vi "read correction factor.vi"(8 "error in (no error)":errorcluster, 11 "Path":path=path "C:/labview project/PSA SubVIs/temp file/trace.csv") -> (0 "error out":errorcluster, 1 "Output Array":dbl[][](array[numeric]), 2 "Number of Columns":i32, 3 "Number of Rows":i32)   [LabVIEW 2016]
doc: "Transfer N*2 (transducer factor) or N*3(limit line file) CSV file to 2D Array, output number of rows and columns as well, so in next module these information can be fomat into strings of SCPI commnad which will be written into PSA through for loop one by one (per frequency list)"
uses:
  <vilib>/Utility/file.llb/Read Delimited Spreadsheet (DBL).vi
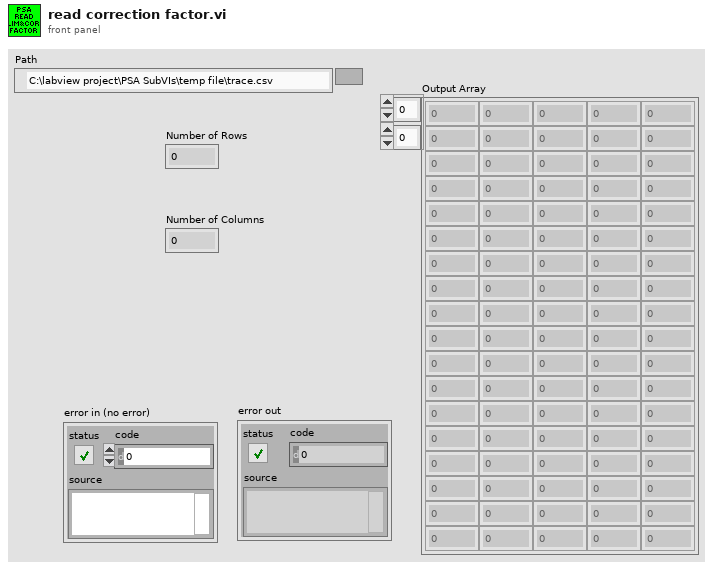
[diagram p1: front panel]
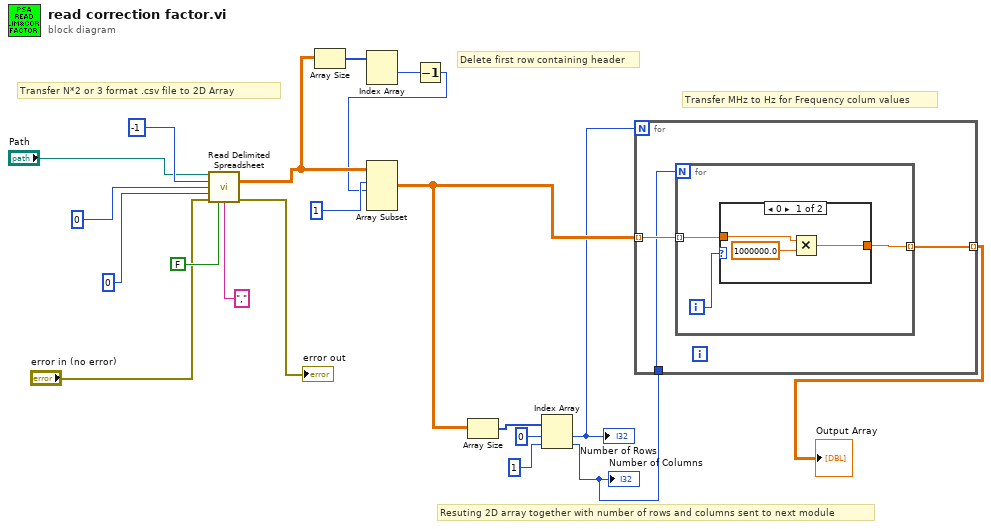
[diagram p0: block diagram]
diagram:
  # "Transfer MHz to Hz for Frequency colum values"
  # "Resuting 2D array together with number of rows and columns sent to next module"
  # "Delete first row containing header"
  # "Transfer N*2 or 3 format .csv file to 2D Array"
  n1 = call-poly <vilib>:"Read Delimited Spreadsheet.vi"("file path (dialog if empty)"="Path", "number of rows (all:-1)"=-1, "start of read offset (chars.:0)"=0, "max characters/row  (no limit:0)"=0, "error in (no error)"="error in (no error)", "transpose? (F)"=FALSE, "delimiter (\\t)"="," ("delimiter (\\t)")) -> ("all rows"=w8:dbl[][], "error out"=→"error out":errorcluster)  [unwired: 3 in, 4 out]
  n2 = Array Size(array=w8) -> (size(s)=w7:i32[])
  n3 = Index Array(array=w7) -> (element #1=w6:i32)  [unwired: 2 in, 1 out]
  n4 = Decrement(x=w6) -> (x-1=w5:i32)
  n5 = Array Subset(array=w8, index (row)=1 ("index"), length (row)=w5) -> (w4:dbl[][])  [unwired: 2 in]
  n6 = Array Size(array=w4) -> (size(s)=w14:i32[])
  n7 = Index Array(array=w14, index #1=0 ("index"), index #2=1 ("index")) -> (element #1=w2:i32, element #2=w1:i32)
  "Number of Columns" <- w1
  "Number of Rows" <- w2
  n8 = for {
    N: w2 -> [_]
    tunnel: w4 -> [w23] mode=indexing
    tunnel: [w22] -> w3 mode=indexing
    tunnel: w1 -> [w21]
    n9 = for {
      N: w21 -> [_]
      tunnel: w23 -> [w26] mode=indexing
      tunnel: [w25] -> w22 mode=indexing
      i -> [w24]
      n10 = case shown="0" w24 {
        tunnel: w26 -> [w28 w30]
        tunnel: [w27 w30] -> w25
        frame 0 {
          n11 = Multiply(x=w28, y=1000000.0) -> (x*y=w27:dbl)
        }
        frame 1, Default {
        }
      }
    }
  }
  "Output Array" <- w3
